vi "Toggle.vi"(1 "in":bool=TRUE) -> (0 "Out":bool=TRUE)   [LabVIEW 2016]
uses:
  <vilib>/functionblocks/Edge Detection/One Shot Rising with Input/One Shot Rising with Input.vi
  <vilib>/functionblocks/FB Core/FB Core.xnode
  <vilib>/functionblocks/NI_FunctionBlock Libraries.lvlib
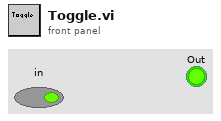
[diagram p1: front panel]
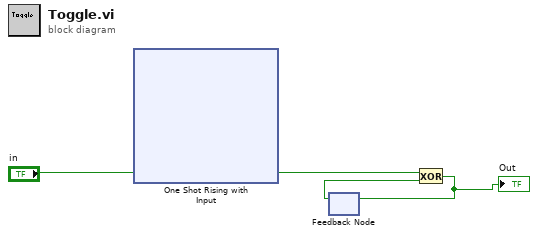
[diagram p0: block diagram]
diagram:
  n1 = xnode "One Shot Rising with Input"("input"="in") -> ("output"=w4:bool)  [unwired: 1 in, 1 out]
  n2 = feedback #1() -> (w3:bool)  [unwired: 1 in]
  n3 = Exclusive Or(1:w3, 2:w4) -> (0:w1:bool)
  "Out" <- w1
  n4 = feedback-in #1(w1) -> ()
